vi "Strip Extension.vi"(10 "Name with Extension":string) -> (2 "Name without Extension":string)   [LabVIEW 2021, in "_Rename.lvlib" / "_Rename.lvclass"]
uses:
  _Rename.lvclass
  _Rename.lvclass/_Rename.ctl
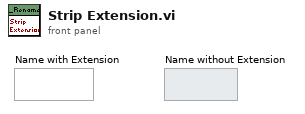
[diagram p1: front panel]
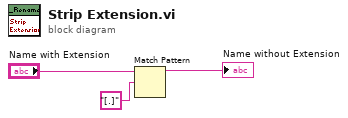
[diagram p0: block diagram]
diagram:
  n1 = Match Pattern(string="Name with Extension", regular expression="[.]") -> (before substring=→"Name without Extension":string)  [unwired: 1 in, 3 out]
